vi "SM_CaseErase.vi"(8 "Input":string[](array[string])) -> (0 "Output":string[](array[string]))   [LabVIEW 2022 SP3]
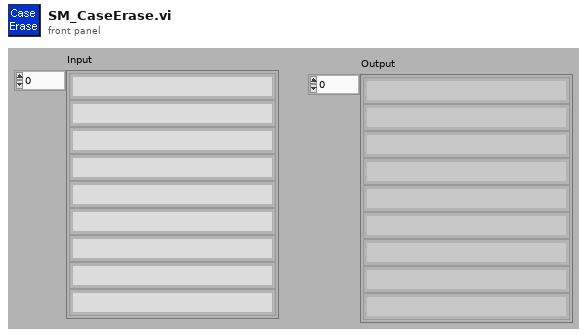
[diagram p1: front panel]
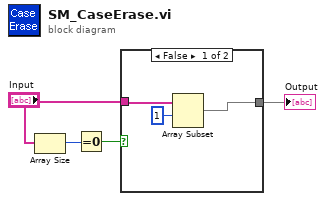
[diagram p0: block diagram]
diagram:
  n1 = Array Size(array="Input") -> (size(s)=w3:i32)
  n2 = Equal To 0?(x=w3) -> (x = 0?=w2:bool)
  n3 = case shown="False" w2 {
    tunnel: "Input" -> [w7 w8]
    tunnel: [w5 w8] -> w1
    frame False {
      n4 = Array Subset(array=w7, index=1 ("指標")) -> (w5:string[])  [unwired: 1 in]
    }
    frame True {
    }
  }
  "Output" <- w1
